vi "RemoveInvalidCharacters.vi"(11 "string in":string) -> (3 "string out":string)   [LabVIEW 2018, in "Python.lvclass"]
uses:
  Python.lvclass
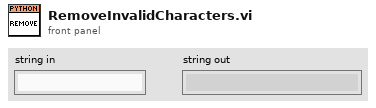
[diagram p1: front panel]
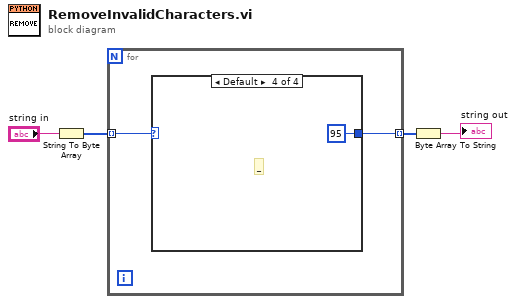
[diagram p0: block diagram]
diagram:
  n1 = String To Byte Array(string="string in") -> (unsigned byte array=w3:u8[])
  n2 = for {
    tunnel: w3 -> [w6] mode=indexing
    tunnel: [w5] -> w2 mode=indexing
    n3 = case shown="Default" w6 {
      selector: w6 -> [w7 w8 w9 _]
      tunnel: [w7 w8 w9 u8 95] -> w5
      frame 48..57 {
        # "0..9"
      }
      frame 65..90 {
        # "A..Z"
      }
      frame 97..122 {
        # "A..Z"
      }
      frame Default {
        # "_"
      }
    }
  }
  n4 = Byte Array To String(unsigned byte array=w2) -> (string=→"string out":string)
